vi "ExSpectGetSlitInfoIN.vi"() -> ()   [LabVIEW 2010]
panel:
  in  "Slit Number":i16=1 min=1 max=4 step=1
  out "Position":dbl format="%.2f"
  out "Speed":dbl format="%.2f"
  out "error out":errorcluster
  in  "error in (no error)":errorcluster
  # "ExSpectGetSlitInfoIN.vi (InSpectrum)\nCamera and Spectrometer control of the InSpectrum.  This vi will open both the camera and spectrograph then read the current position and speed of the selected slit."
  # "NOTES:\nA properly configured spectometer .ini must be present in the LabVIEW folder for spectrograph operation.\n\nConsult the Toolkit documentation for more information on how to configure this file."
  # "um"
  # "1 = Front Entrance\n 2 = Side Entrance\n 3 = Front Exit\n 4 = Side Exit"
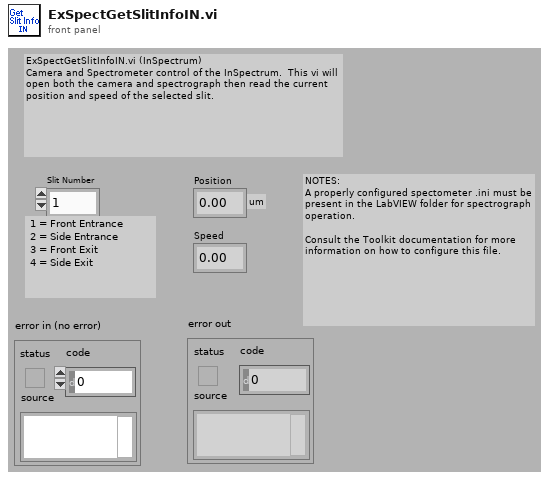
[diagram p1: front panel]
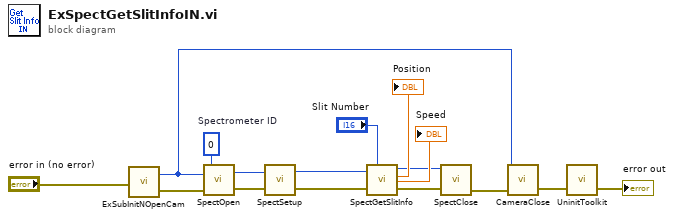
[diagram p0: block diagram]
diagram:
  w13 = u32 0  # Spectrometer ID
  n1 = call "ExSubInitNOpenCam.vi"("error in (no error)"="error in (no error)") -> ("Camera Handle"=w1:u32, "error out"=w12:errorcluster)
  n2 = call <userlib>:"SpectOpen.vi"("error in"=w12, "Camera Handle"=w1, "Spectrometer ID"=w13) -> ("error out"=w14:errorcluster, "Spectrometer Handle"=w15:u32)
  n3 = call <userlib>:"SpectSetup.vi"("error in"=w14, "Spectrometer Handle"=w15) -> ("error out"=w7:errorcluster, "Spectrometer Handle"=w8:u32)
  n4 = call <userlib>:"SpectGetSlitInfo.vi"("Spectrometer Handle"=w8, "Slit"="Slit Number", "error in"=w7) -> ("Spectrometer Handle"=w2:u32, "Position"=→"Position":dbl, "Speed"=→"Speed":dbl, "error out"=w6:errorcluster)
  n5 = call <userlib>:"SpectClose.vi"("error in"=w6, "Spectrometer Handle"=w2) -> ("error out"=w5:errorcluster)
  n6 = call <userlib>:"CameraClose.vi"("error in"=w5, "Camera Handle"=w1) -> ("error out"=w4:errorcluster)
  n7 = call <userlib>:"UninitToolkit.vi"("error in"=w4) -> ("error out"=→"error out":errorcluster)
